vi "Reset VI.vi"(8 "error in (no error)":errorcluster, 9 "Template":refnum<vi>, 10 "Destination":refnum<vi>) -> (0 "error out":errorcluster)   [LabVIEW 2015, in "Message Maker.lvclass"]
doc: "Deletes all elements on the front panel and block diagram. Then it copies the contents from the source VI, and makes the connector panes match\n\nAuthor: Derek Trepanier\nCopyright: MGI 2015"
uses:
  Message Maker.lvclass
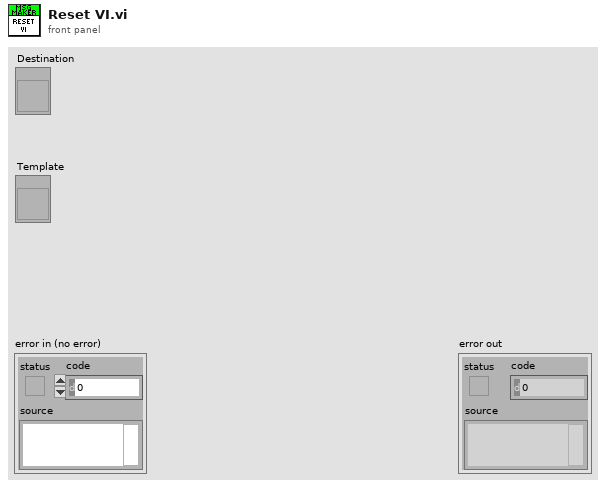
[diagram p1: front panel]
types:
  T1 = enum16{"Share clones between instances", "Preallocate clone for each instance"}
  T2 = enum16{"Invalid Wire Rule", "Required", "Recommended", "Optional", "Dynamic Dispatch"}[]
  T3 = typedef "LVPositionTypeDef.ctl" = cluster{"Left":i32, "Top":i32}
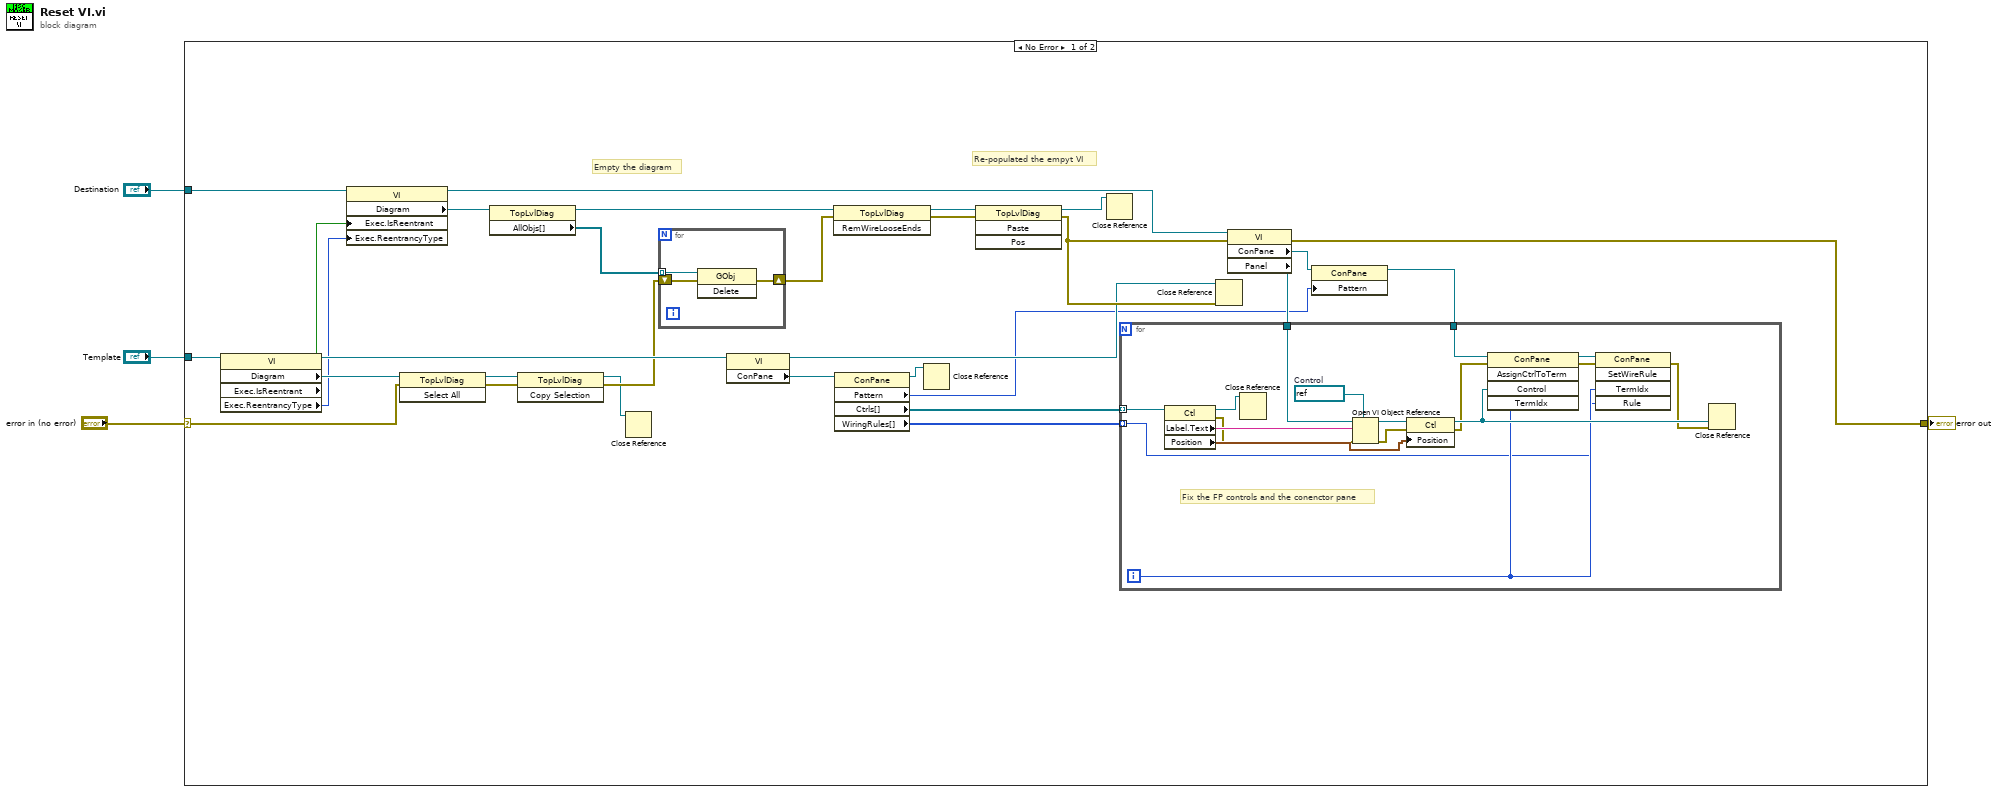
[diagram p0: block diagram]
diagram:
  n1 = case shown="No Error" "error in (no error)" {
    selector: "error in (no error)" -> [w11 w55]
    tunnel: [w12 w55] -> w3
    tunnel: "Destination" -> [w20 _]
    tunnel: "Template" -> [w19 _]
    frame No Error {
      # "Re-populated the empyt VI"
      # "Empty the diagram"
      n2 = property class="VI"(reference=w19) -> (reference out=w24:refnum<vi>, "Diagram"=w34:refnum<vi>, "Exec.IsReentrant"=w6:bool, "Exec.ReentrancyType"=w5:T1)  [unwired: 1 in, 1 out]
      n3 = property class="VI"(reference=w20, "Exec.IsReentrant"=w6, "Exec.ReentrancyType"=w5) -> (reference out=w25:refnum<vi>, "Diagram"=w32:refnum<vi>)  [unwired: 1 in, 1 out]
      n4 = invoke class="TopLvlDiag" method="Select All"(reference=w34, error in=w11) -> (reference out=w33:refnum<vi>, error out=w17:errorcluster)  [unwired: 1 in, 1 out]
      n5 = property class="TopLvlDiag"(reference=w32) -> (reference out=w27:refnum<vi>, "AllObjs[]"=w31:refnum<vi>[])  [unwired: 1 in, 1 out]
      n6 = invoke class="TopLvlDiag" method="Copy Selection"(reference=w33, error in=w17) -> (reference out=w13:refnum<vi>, error out=w18:errorcluster)  [unwired: 1 in, 1 out]
      n7 = Close Reference(reference=w13) -> ()  [unwired: 1 in, 1 out]
      n8 = for {
        tunnel: w31 -> [w54] mode=indexing
        shift-right: [w53] -> w30
        shift-left: w18 -> [w52]
        n9 = invoke class="GObj" method="Delete"(reference=w54, error in=w52) -> (error out=w53:errorcluster)  [unwired: 1 in, 2 out]
      }
      n10 = property class="VI"(reference=w24) -> (reference out=w16:refnum<vi>, "ConPane"=w23:refnum<vi>)  [unwired: 1 in, 1 out]
      n11 = invoke class="TopLvlDiag" method="RemWireLooseEnds"(reference=w27, error in=w30) -> (reference out=w28:refnum<vi>, error out=w29:errorcluster)  [unwired: 1 in, 1 out]
      n12 = property class="ConPane"(reference=w23) -> (reference out=w15:refnum<vi>, "Pattern"=w8:u32, "Ctrls[]"=w21:refnum<vi>[], "WiringRules[]"=w10:T2)  [unwired: 1 in, 1 out]
      n13 = Close Reference(reference=w15) -> ()  [unwired: 1 in, 1 out]
      n14 = invoke class="TopLvlDiag" method="Paste"(reference=w28, error in=w29) -> (reference out=w14:refnum<vi>, error out=w26:errorcluster)  [unwired: 2 in, 2 out]
      n15 = Close Reference(reference=w14) -> ()  [unwired: 1 in, 1 out]
      n16 = Close Reference(reference=w16, error in (no error)=w26) -> ()  [unwired: 1 out]
      n17 = property class="VI"(reference=w25, error in=w26) -> (error out=w12:errorcluster, "ConPane"=w9:refnum<vi>, "Panel"=w22:refnum<vi>)  [unwired: 1 out]
      n18 = property class="ConPane"(reference=w9, "Pattern"=w8) -> (reference out=w7:refnum<vi>)  [unwired: 1 in, 1 out]
      n19 = for {
        tunnel: w22 -> [w51]
        tunnel: w21 -> [w49] mode=indexing
        tunnel: w10 -> [w36] mode=indexing
        tunnel: w7 -> [w42]
        i -> [w37]
        w50 = refnum<vi> refnum  # Control
        # "Fix the FP controls and the conenctor pane"
        n20 = property class="Ctl"(reference=w49) -> (reference out=w45:refnum<vi>, error out=w44:errorcluster, "Label.Text"=w48:string, "Position"=w46:T3)  [unwired: 1 in]
        n21 = Close Reference(reference=w45) -> ()  [unwired: 1 in, 1 out]
        n22 = Open VI Object Reference(7:w50, 8:w44, 10:w48, 11:w51) -> (0:w43:errorcluster, 3:w47:refnum<vi>)
        n23 = property class="Ctl"(reference=w47, error in=w43, "Position"=w46) -> (reference out=w41:refnum<vi>, error out=w40:errorcluster)
        n24 = invoke class="ConPane" method="AssignCtrlToTerm"(reference=w42, error in=w40, "Control"=w41, "TermIdx"=w37) -> (reference out=w39:refnum<vi>, error out=w38:errorcluster)  [unwired: 1 in, 3 out]
        n25 = invoke class="ConPane" method="SetWireRule"(reference=w39, error in=w38, "TermIdx"=w37, "Rule"=w36) -> (error out=w35:errorcluster)  [unwired: 1 in, 4 out]
        n26 = Close Reference(reference=w41, error in (no error)=w35) -> ()  [unwired: 1 out]
      }
    }
    frame Error {
    }
  }
  "error out" <- w3
